vi "Init Digital Input.vi"(9 "DIO Channel":T2, 10 "Digital Module":T3, 11 "Refnum":string) -> (3 "DigitalInputDevRef":T1={"DevStatus"={"status"=FALSE, "code"=0, "source"=""}, "DIO Channel"=enum."Invalid", "Digital Module"=enum."Digital Module 1"})   [LabVIEW 2012]
uses:
  <vilib>/Rock Robotics/SystemInterfaces/DIO/FPGA_DIOChannel.ctl
  <vilib>/Rock Robotics/SystemInterfaces/Typedef/FPGA_TypedefDigitalModule.ctl
  <vilib>/Rock Robotics/WPI/DigitalInput/WPI_DigitalInputDevRef.ctl
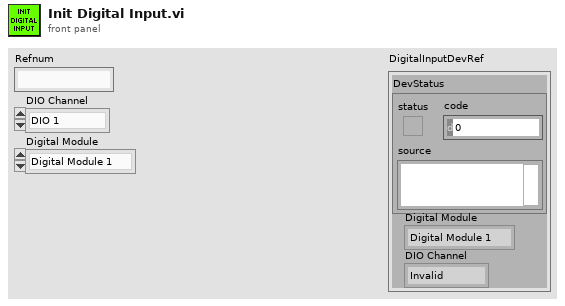
[diagram p1: front panel]
types:
  T1 = typedef "WPI_DigitalInputDevRef.ctl" = cluster{"DevStatus":errorcluster, "DIO Channel":T2, "Digital Module":T3}
  T2 = typedef "FPGA_DIOChannel.ctl" = enum8{"DIO 1", "DIO 2", "DIO 3", "DIO 4", "DIO 5", "DIO 6", "DIO 7", "DIO 8", "DIO 9", "DIO 10", "DIO 11", "DIO 12", "DIO 13", "DIO 14", "Invalid"}
  T3 = typedef "FPGA_TypedefDigitalModule.ctl" = enum16{"Digital Module 1", "Digital Module 2"}
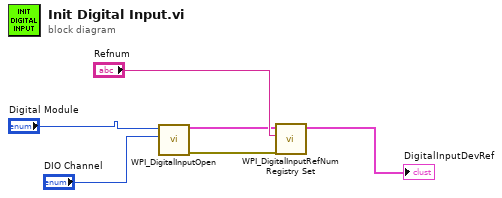
[diagram p0: block diagram]
diagram:
  n1 = call <vilib>:"WPI_DigitalInputOpen.vi"("DIO Channel"="DIO Channel", "Digital Module (Module 1)"="Digital Module") -> ("error out"=w4:errorcluster, "DigitalInputDevRef"=w5:T1)  [unwired: 8 in]
  n2 = call <vilib>:"WPI_DigitalInputRefNum Registry Set.vi"("error in (no error)"=w4, "refnum name"="Refnum", "DigitalInputDevRef"=w5) -> ("DigitalInputDevRef"=→"DigitalInputDevRef":T1)  [unwired: 7 in, 1 out]
